vi "PlotDailies.vi"() -> ()   [LabVIEW 2019]
uses:
  <userlib>/LevyLab/XY Utilities/subVIs/Append (double array).vi
  <userlib>/LevyLab/XY Utilities/subVIs/Get X and Y (single).vi
  <userlib>/_OpenG.lib/array/array.llb/Sort 1D Array (DBL)__ogtk.vi
  <userlib>/_OpenG.lib/array/array.llb/Reorder 1D Array2 (Path)__ogtk.vi
  <userlib>/LevyLab/Graph Utilities/graph_utilities.lvclass
  <userlib>/LevyLab/XY Utilities/xy_utilities.lvlib
panel:
  in  "items":i32[](listbox)
  in  "files":i32[](listbox)
  out "XY Graph":cluster{dbl[], dbl[]}[](graph)
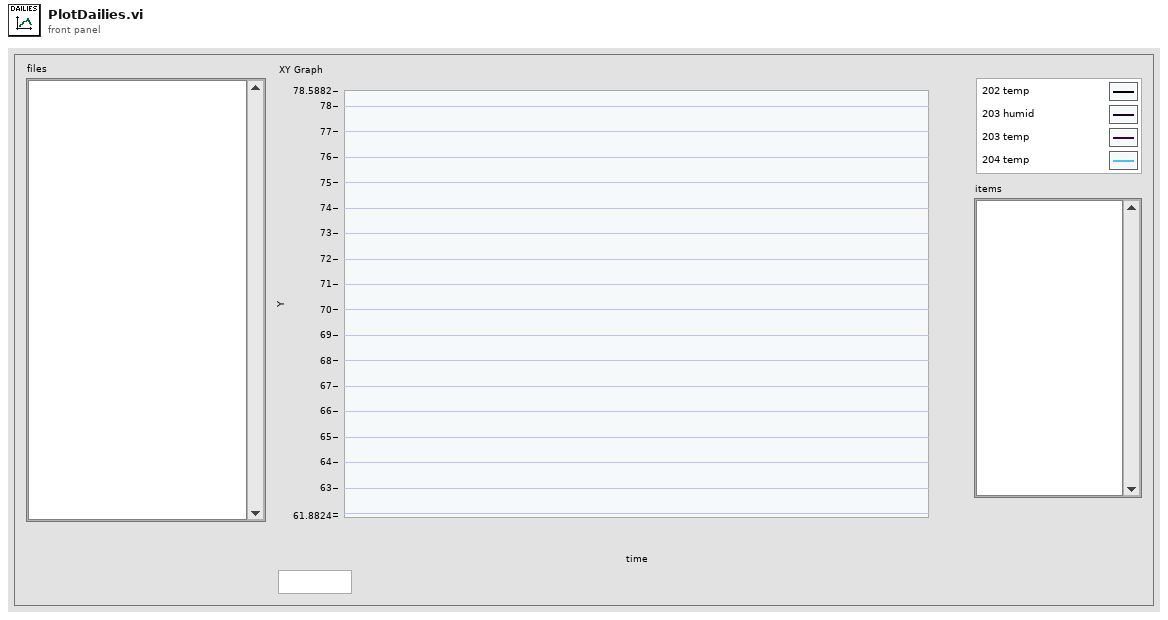
[diagram p1: front panel]
types:
  T1 = enum32{"Invalid", "Standard", "Closed", "Hidden", "Minimized", "Maximized"}
  T2 = enum32{"invalid app kind", "Development System", "Run Time System", "Student Edition", "Embedded LabVIEW", "Evaluation", "Custom"}
  T3 = enum16{"CET-C1", "CET-C1s", "CET-C2", "CET-C2s", "CET-C3", "CET-C3s", "CET-C4", "CET-C4s", "CET-C5", "CET-C5s", "CET-C6", "CET-C6s", "CET-C7", "CET-C7s", "CET-CBC1", "CET-CBC2", "CET-CBD1", "CET-CBL1", "CET-CBL2", "CET-D01", "CET-D01A", "CET-D02", "CET-D03", "CET-D04", "CET-D06", "CET-D07", "CET-D08", "CET-D09", "CET-D10", "CET-D11", "CET-D12", "CET-D13", "CET-I1", "CET-I2", "CET-I3", "CET-L01", "CET-L02", "CET-L03", "CET-L04", "CET-L05", "CET-L06", "CET-L07", "CET-L08", "CET-L09", "CET-L10", "CET-L11", "CET-L12", "CET-L13", "CET-L14", "CET-L15", "CET-L16", "CET-L17", "CET-L18", "CET-L19", "CET-L20", "CET-R1", "CET-R2", "CET-R3", "CET-R4"}
  T4 = enum16{"Inferno", "Kindlmann", "Plasma", "Viridis", "LevyLab2010", "ColorCET...", "Custom..."}
  T5 = cluster{"Core":cluster{"Current VI Reference":refnum<vi>, "Close Panel on Exit?":bool}, "dailies folder":path, "file paths":path[], "file path":path, "items":string[], "Map":map{string, dbl[]}, "XY-data":cluster{"X-array":dbl[], "Y-array":dbl[]}[]}
  T6 = cluster{"Current VI Reference":refnum<vi>, "Close Panel on Exit?":bool}
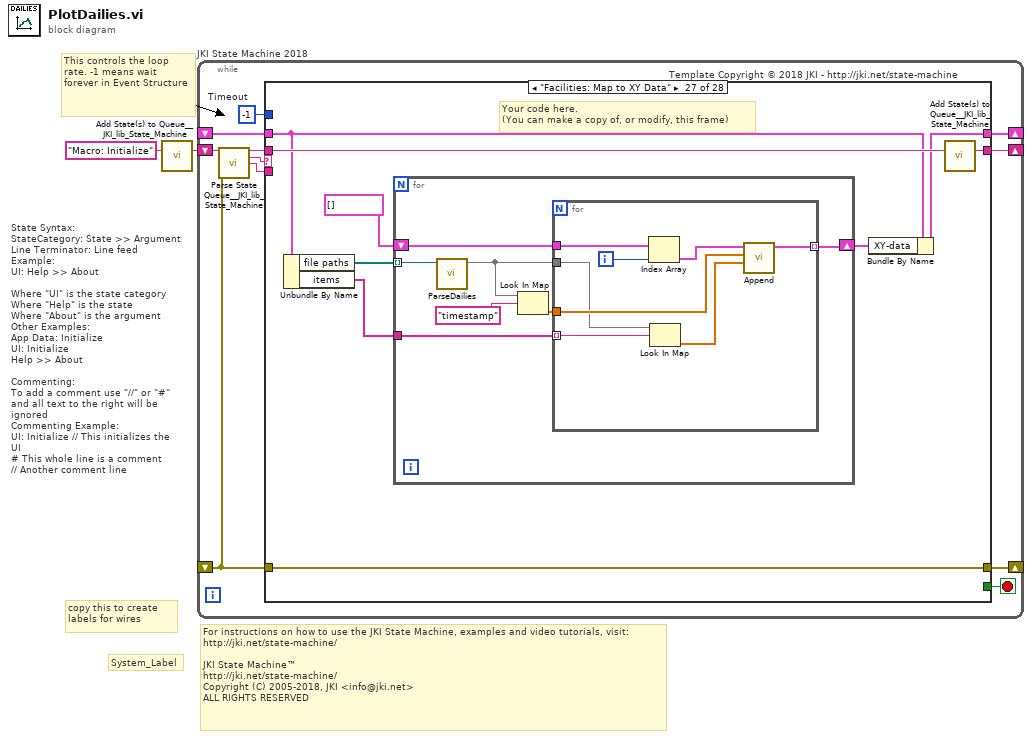
[diagram p0: block diagram]
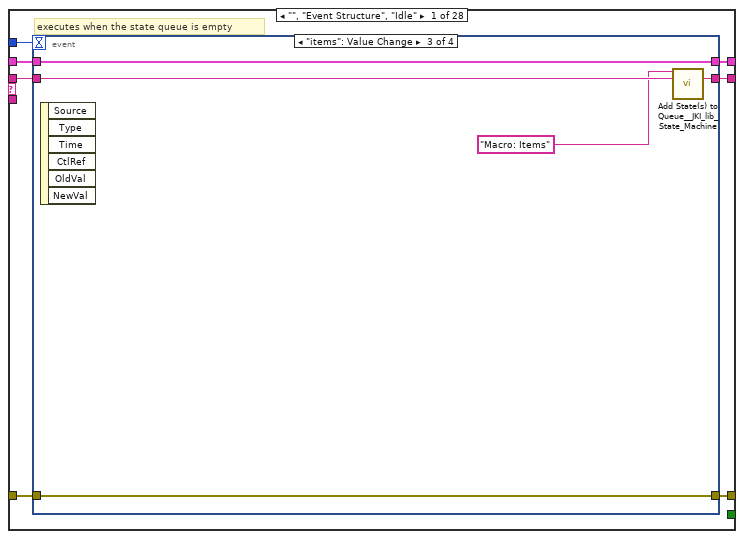
[diagram p2: hidden frame]
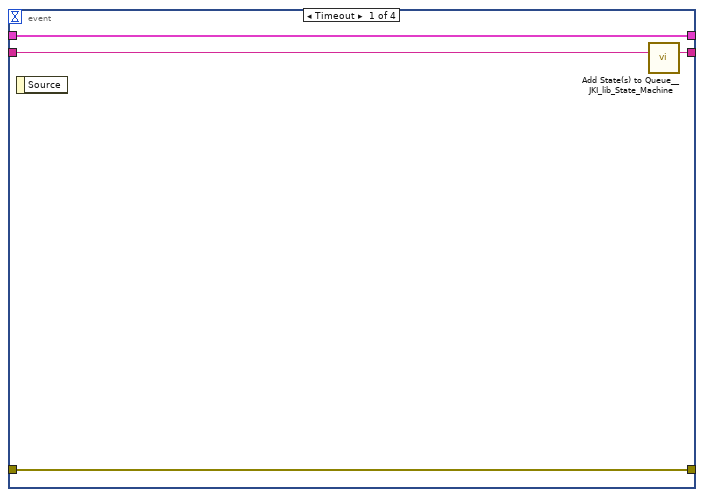
[diagram p3: hidden frame]
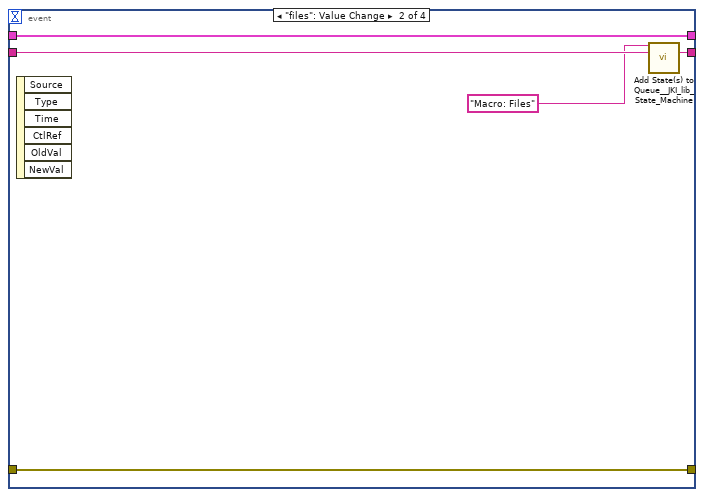
[diagram p4: hidden frame]
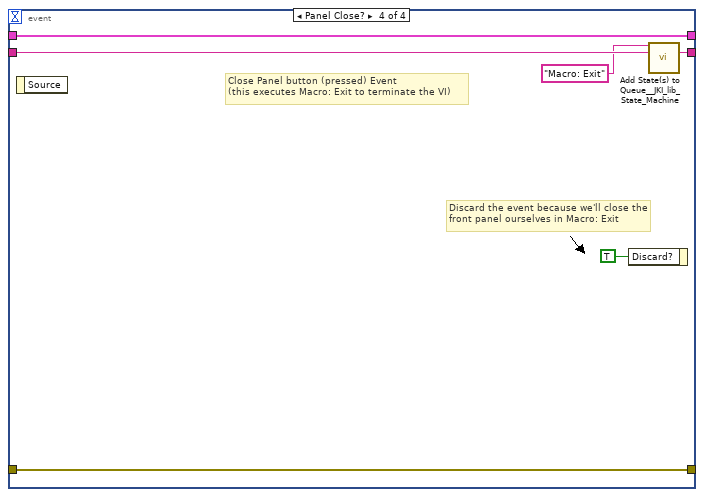
[diagram p5: hidden frame]
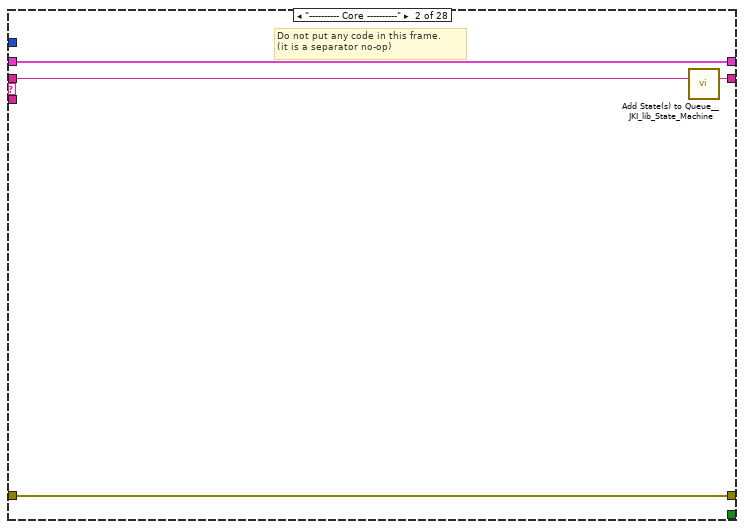
[diagram p6: hidden frame]
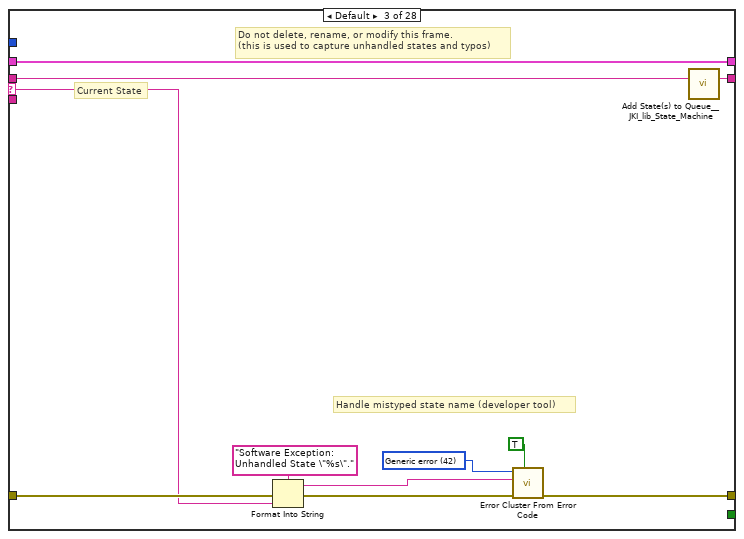
[diagram p7: hidden frame]
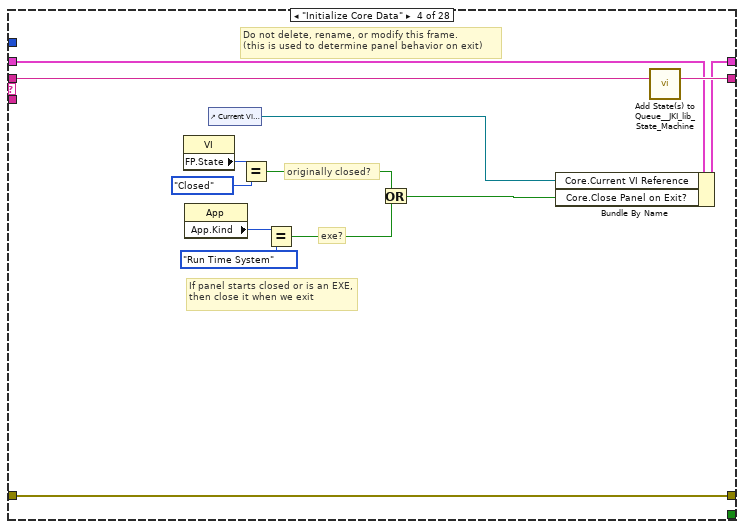
[diagram p8: hidden frame]
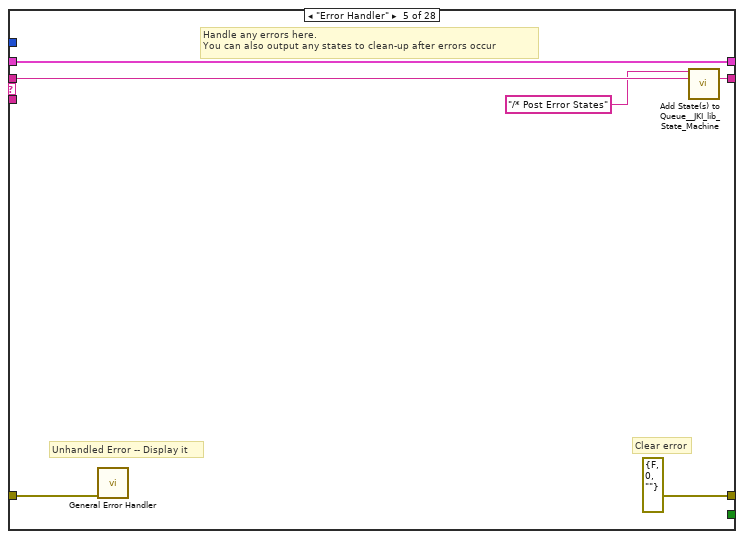
[diagram p9: hidden frame]
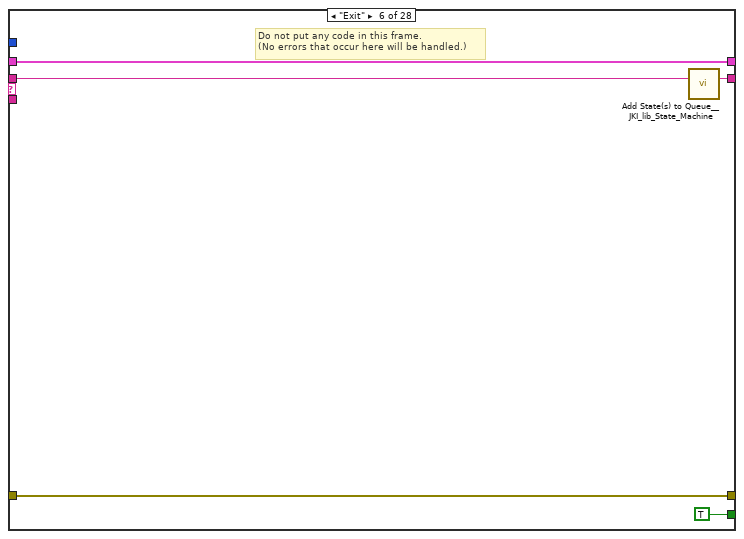
[diagram p10: hidden frame]
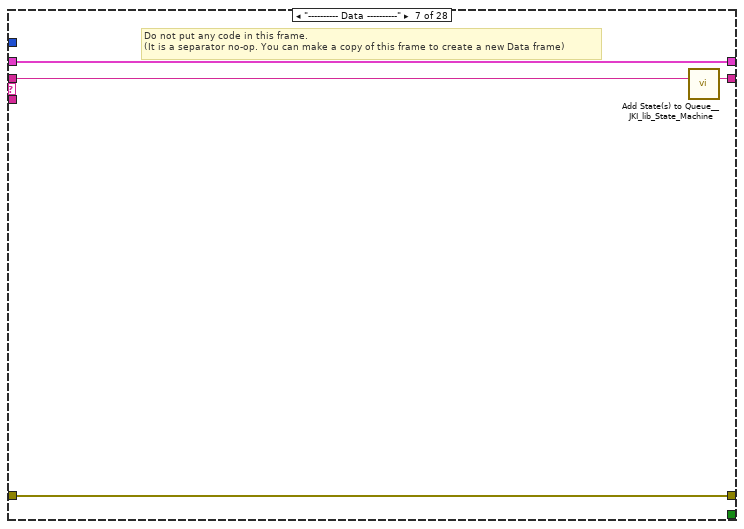
[diagram p11: hidden frame]
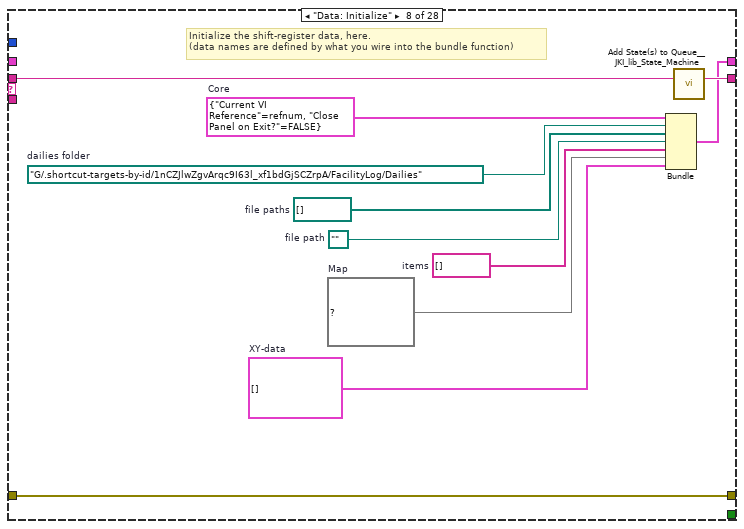
[diagram p12: hidden frame]
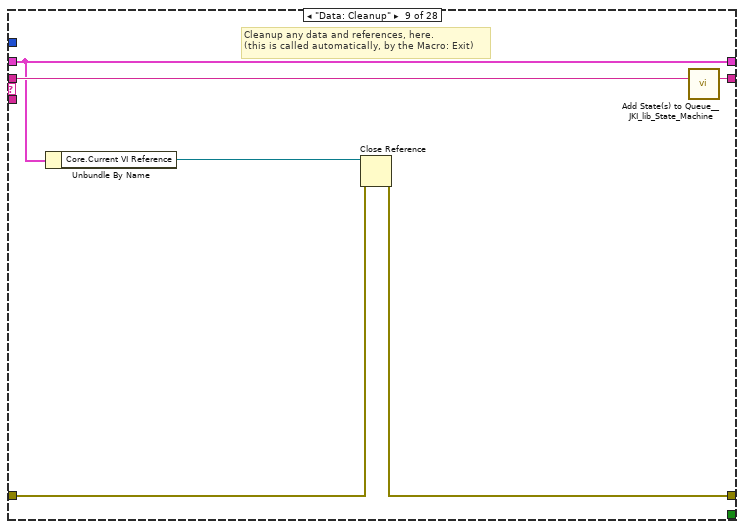
[diagram p13: hidden frame]
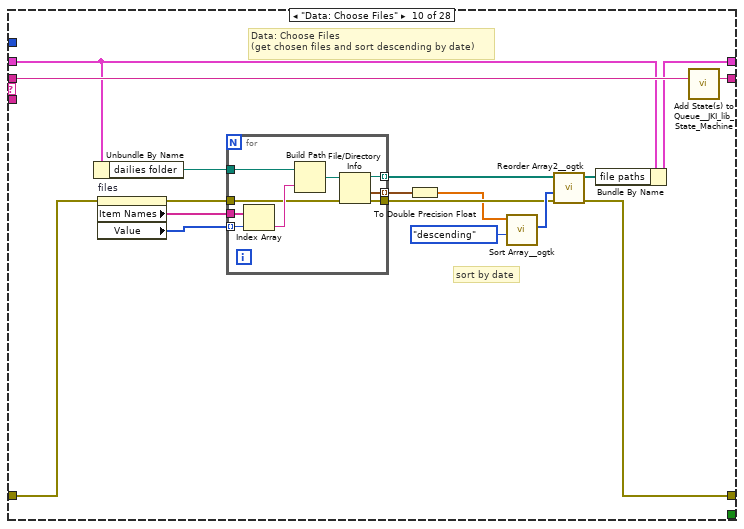
[diagram p14: hidden frame]
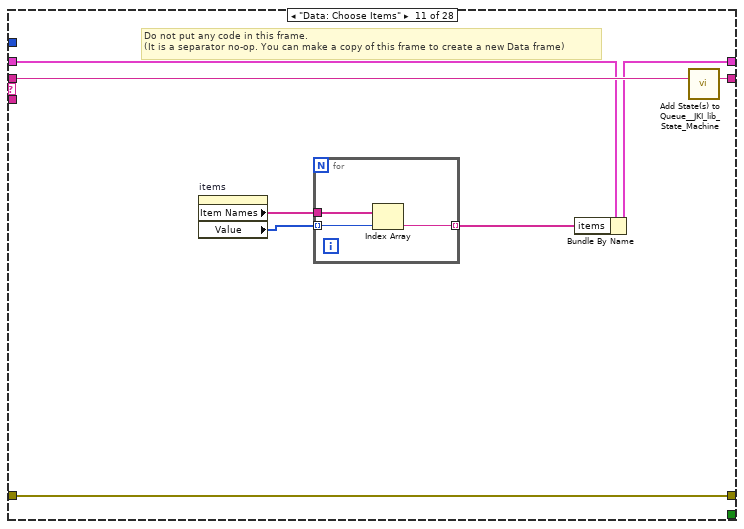
[diagram p15: hidden frame]
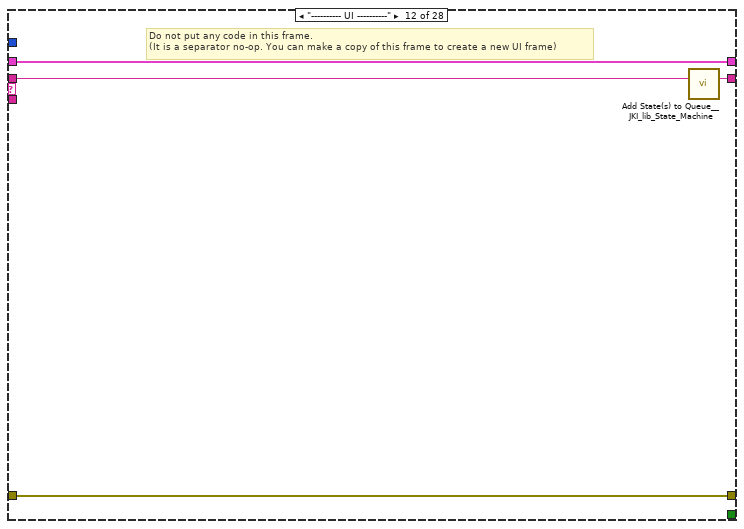
[diagram p16: hidden frame]
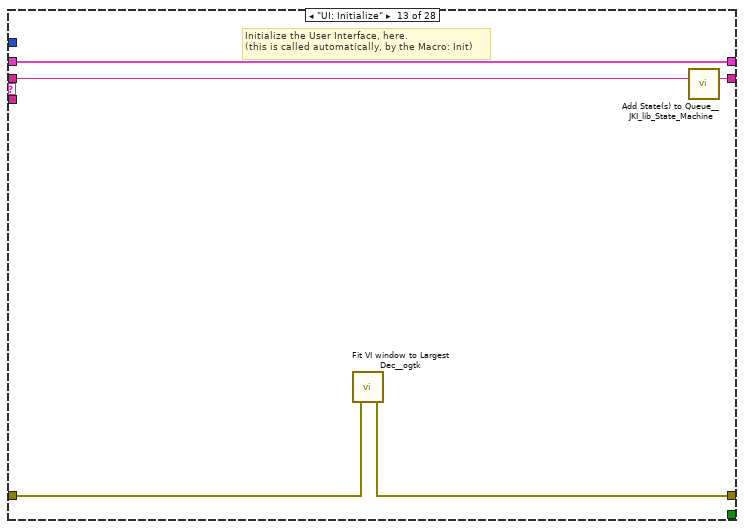
[diagram p17: hidden frame]
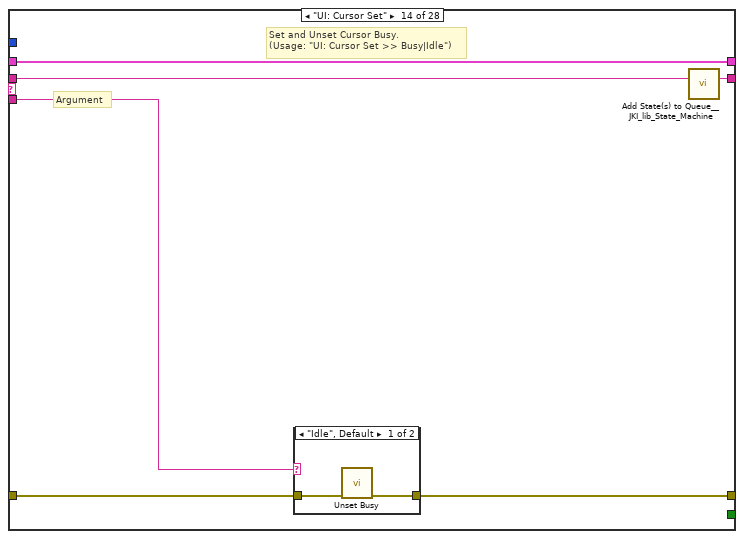
[diagram p18: hidden frame]
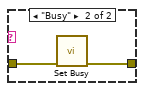
[diagram p19: hidden frame]
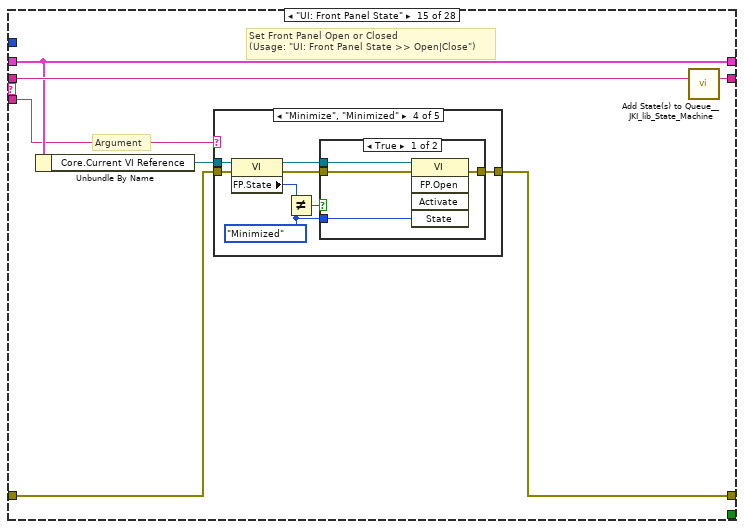
[diagram p20: hidden frame]
diagram:
  # "For instructions on how to use the JKI State Machine, examples and video tutorials, visit:\nhttp://jki.net/state-machine/\n\nJKI State Machine™\nhttp://jki.net/state-machine/\nCopyright (C) 2005-2018, JKI <info@jki.net>\nALL RIGHTS RESERVED"
  # "State Syntax:\nStateCategory: State >> Argument\nLine Terminator: Line feed\nExample:\nUI: Help >> About\n\nWhere \"UI\" is the state category\nWhere \"Help\" is the state\nWhere \"About\" is the argument\nOther Examples:\nApp Data: Initialize\nUI: Initialize\nHelp >> About\n\nCommenting:\nTo add a comment use \"//\" or \"#\" and all text to the right will be ignored\nCommenting Example:\nUI: Initialize // This initializes the UI\n# This whole line is a comment\n// Another comment line"
  # "copy this to create labels for wires"
  # "This controls the loop rate. -1 means wait forever in Event Structure"
  # "System_Label"
  n1 = call <vilib>:"Add State(s) to Queue__JKI_lib_State_Machine.vi"("State(s) in (\"\")"="Macro: Initialize") -> ("States Out"=w2:string)  [unwired: 14 in]
  n2 = while "JKI State Machine 2018" {
    shift-right: [w6] -> _
    shift-left: _ -> [w5]
    shift-right: [w9] -> _
    shift-left: _ -> [w3]
    shift-right: [w8] -> _
    shift-left: w2 -> [w10]
    stop <- w7 stop-if-true
    w4 = -1  # Timeout
    # "Template Copyright © 2018 JKI - http://jki.net/state-machine"
    n3 = call <vilib>:"Parse State Queue__JKI_lib_State_Machine.vi"("State Queue"=w10, "Error In (no error)"=w3) -> ("Remaining States"=w12:string, "Current State"=w13:string, "Arguments"=w11:string)  [unwired: 11 in]
    n4 = case shown="\"Facilities: Map to XY Data\"" w13 {
      selector: w13 -> [_ _ w45 _ _ _ _ _ _ _ _ _ _ _ _ _ _ _ _ _ _ _ _ _ _ _ _ _]
      tunnel: w12 -> [w20 w44 w49 w68 w74 w79 w83 w94 w100 w116 w133 w140 w145 w151 w162 w238 w244 w264 w278 w282 w288 w298 w309 w314 w318 w327 w336 w365]
      tunnel: w11 -> [_ _ _ _ _ _ _ _ _ _ _ _ _ w146 w156 _ _ _ _ _ _ _ _ _ _ _ _ _]
      tunnel: w5 -> [w18 w41 w47 w61 w71 w77 w80 _ w95 w101 w127 w137 w143 w149 w158 w232 w240 w261 w275 w279 w285 w295 w306 w311 w315 w325 w331 w355]
      tunnel: [w17 w42 w51 w65 errorcluster {"status"=FALSE, "code"=0, "source"=""} ("error out") w76 w81 w91 w96 w106 w131 w138 w142 w147 w159 w235 w242 w262 w276 w280 w286 w296 w307 w312 w316 w322 w334 w352] -> w9
      tunnel: w3 -> [w16 w42 w50 w65 w70 w76 w81 w91 w97 w105 w131 w138 w141 w148 w160 w234 w242 w262 w276 w280 w286 w296 w307 w312 w316 w321 w334 w353]
      tunnel: [w19 w43 w48 w67 w73 w78 w82 w93 w99 w115 w132 w139 w144 w150 w161 w237 w243 w263 w277 w281 w287 w297 w308 w313 w317 w326 w335 w364] -> w8
      tunnel: [_ _ _ _ _ TRUE _ _ _ _ _ _ _ _ _ _ _ _ _ _ _ _ _ _ _ _ _ _] -> w7
      tunnel: [w15 w41 w47 w66 w71 w77 w80 w92 w95 w102 w128 w137 w143 w149 w158 w232 w240 w261 w275 w279 w285 w295 w306 w311 w315 w323 w332 w356] -> w6
      tunnel: w4 -> [w14 _ _ _ _ _ _ _ _ _ _ _ _ _ _ _ _ _ _ _ _ _ _ _ _ _ _ _]
      frame "", "Event Structure", "Idle" {
        # "executes when the state queue is empty"
        n5 = event shown="[2] \"items\": Value Change" {
          selector: _ -> [_ _ _ _]
          dyn-events: _ -> [_ _ _ _]
          timeout: w14 -> [_ _ _ _]
          tunnel: w20 -> [w24 w29 w34 w40]
          tunnel: [w23 w28 w33 w39] -> w19
          tunnel: w18 -> [w21 w26 w31 w37]
          tunnel: [w22 w27 w32 w38] -> w17
          tunnel: w16 -> [w22 w27 w32 w38]
          tunnel: [w21 w26 w31 w37] -> w15
          event Timeout {
            n6 = event-data() -> ()  [unwired: 1 in, 1 out]
            n7 = call <vilib>:"Add State(s) to Queue__JKI_lib_State_Machine.vi"("State(s) in (\"\")"=w24) -> ("States Out"=w23:string)  [unwired: 14 in]
          }
          event "files": Value Change {
            n8 = event-data() -> ()  [unwired: 1 in, 6 out]
            n9 = call <vilib>:"Add State(s) to Queue__JKI_lib_State_Machine.vi"("State(s) in Front (\"\")"="Macro: Files" ("State(s) in Front (\"\")"), "State(s) in (\"\")"=w29) -> ("States Out"=w28:string)  [unwired: 13 in]
          }
          event "items": Value Change {
            n10 = event-data() -> ()  [unwired: 1 in, 6 out]
            n11 = call <vilib>:"Add State(s) to Queue__JKI_lib_State_Machine.vi"("State(s) in Front (\"\")"="Macro: Items" ("State(s) in Front (\"\")"), "State(s) in (\"\")"=w34) -> ("States Out"=w33:string)  [unwired: 13 in]
          }
          event Panel Close? {
            # "Discard the event because we'll close the front panel ourselves in Macro: Exit"
            # "Close Panel button (pressed) Event\n(this executes Macro: Exit to terminate the VI)"
            n12 = event-data() -> ()  [unwired: 1 in, 1 out]
            n13 = event-data("Discard?"=TRUE) -> ()  [unwired: 1 in, 1 out]
            n14 = call <vilib>:"Add State(s) to Queue__JKI_lib_State_Machine.vi"("State(s) in Front (\"\")"="Macro: Exit", "State(s) in (\"\")"=w40) -> ("States Out"=w39:string)  [unwired: 13 in]
          }
        }
      }
      frame "---------- Core ----------" {
        # "Do not put any code in this frame.\n(it is a separator no-op)"
        n15 = call <vilib>:"Add State(s) to Queue__JKI_lib_State_Machine.vi"("State(s) in (\"\")"=w44) -> ("States Out"=w43:string)  [unwired: 14 in]
      }
      frame Default {
        w54 = 42 items=["No error", "Argument error", "Memory is full", "Out of zone", "End of file", "File already open", "Generic file I/O error", "File not found", "File permission error", "Disk is full", "Duplicate path", "Too many files open", "System feature not enabled", "Resource file not found", "Cannot add resource", "Resource not found", "Image not found", "Image memory error", "Pen does not exist", "Config type invalid", "Config token not found", "Config parse error", "Config memory error", "Bad external code format", "Bad external code offset", "External code not present", "Null window", "Destroy window error", "Null menu", "Print aborted", "Bad print record", "Print driver error", "Windows error during printing", "Memory error during printing", "Print dialog error", "Generic print error", "Invalid device refnum", "Device not found", "Device parameter error", "Device unit error", "Cannot open device", "Device call aborted", "Generic error", "Cancelled by user", "Object ID too low", "Object ID too high", "Object not in heap", "Unknown heap", "Unknown object (invalid DefProc)", "Unknown object (DefProc not in table)", "Message out of range", "Invalid (null) method", "Unknown message", "Manager call not supported", "Bad address", "Network operation in progress", "Network operation timed out", "Connection is busy", "Network attribute not supported", "Network error", "Address in use", "System out of memory", "Connection aborted", "Connection refused", "Not connected", "Already connected", "Connection closed", "Initialization error (interapplication manager)", "Bad occurrence", "Wait on unbound occurrence handler", "Occurrence queue overflow", "Datalog type conflict", "Unused", "Unrecognized type (interapplication manager)", "Memory corrupt", "Failed to make temporary DLL", "Old CIN version", "Drag socket not found", "Failed to load drop-object", "Failed to register OLE object", "Failed to release OLE object", "Format specifier type mismatch", "Unknown format specifier", "Too few format specifiers", "Too many format specifiers", "Scan failed", "Newer CIN version", "Error converting to variant", "Runtime menu error", "Password tampered", "Variant attribute not found", "Incompatible variant data type", "Event data is not available", "Event Store is not present", "Occurrence is not found", "Event Queue is not created", "Event info is not available", "Refnum passed is NULL", "Error retrieving Class GUID", "Error retrieving CoClass GUID", "Error retrieving TypeLib GUID.", "Bad built application magic bytes.", "Specific driver is different from the specific driver associated with the Logical Name.", "There is no session opened to the class driver.", "Max Error", "MAX - Error with config objects", "MAX - Error loading configuration", "MAX - Group not supported"]
        # "Current State"
        # "Do not delete, rename, or modify this frame.\n(this is used to capture unhandled states and typos)"
        # "Handle mistyped state name (developer tool)"
        n16 = Format Into String(format string="Software Exception: Unhandled State \"%s\"." ("message"), error in=w50, w45) -> (resulting string=w53:string, error out=w52:errorcluster)  [unwired: 1 in]
        n17 = call <vilib>:"Error Cluster From Error Code.vi"("show call chain? (False)"=TRUE, "error in (no error)"=w52, "error message (\"\")"=w53, "error code (0)"=w54) -> ("error out"=w51:errorcluster)  [unwired: 5 in]
        n18 = call <vilib>:"Add State(s) to Queue__JKI_lib_State_Machine.vi"("State(s) in (\"\")"=w49) -> ("States Out"=w48:string)  [unwired: 14 in]
      }
      frame "Initialize Core Data" {
        # "Do not delete, rename, or modify this frame.\n(this is used to determine panel behavior on exit)"
        # "originally closed?"
        # "exe?"
        # "If panel starts closed or is an EXE, then close it when we exit"
        n19 = property class="VI"() -> ("FP.State"=w58:T1)  [unwired: 2 in, 2 out]
        n20 = property class="App"() -> ("App.Kind"=w64:T2)  [unwired: 2 in, 2 out]
        n21 = control-ref of="Current VI Reference"() -> (w59:refnum<vi>)
        n22 = Equal?(x=w58, y=T1."Closed" ("Front Panel Window:State")) -> (x = y?=w56:bool)
        n23 = Equal?(x=w64, y=T2."Run Time System" ("Application:Kind")) -> (x = y?=w62:bool)
        n24 = Or(x=w56, y=w62) -> (x .or. y?=w60:bool)
        n25 = Bundle By Name(cluster=w61, "Core.Current VI Reference"=w59, "Core.Close Panel on Exit?"=w60) -> (w66:T5)
        n26 = call <vilib>:"Add State(s) to Queue__JKI_lib_State_Machine.vi"("State(s) in (\"\")"=w68) -> ("States Out"=w67:string)  [unwired: 14 in]
      }
      frame "Error Handler" {
        # "Unhandled Error -- Display it"
        # "Handle any errors here.\nYou can also output any states to clean-up after errors occur"
        # "Clear error"
        n27 = call <vilib>:"General Error Handler.vi"("error in (no error)"=w70) -> ()  [unwired: 10 in, 5 out]
        n28 = call <vilib>:"Add State(s) to Queue__JKI_lib_State_Machine.vi"("State(s) in Front (\"\")"="/* Post Error States", "State(s) in (\"\")"=w74) -> ("States Out"=w73:string)  [unwired: 13 in]
      }
      frame "Exit" {
        # "Do not put any code in this frame.\n(No errors that occur here will be handled.)"
        n29 = call <vilib>:"Add State(s) to Queue__JKI_lib_State_Machine.vi"("State(s) in (\"\")"=w79) -> ("States Out"=w78:string)  [unwired: 14 in]
      }
      frame "---------- Data ----------" {
        # "Do not put any code in this frame.\n(It is a separator no-op. You can make a copy of this frame to create a new Data frame)"
        n30 = call <vilib>:"Add State(s) to Queue__JKI_lib_State_Machine.vi"("State(s) in (\"\")"=w83) -> ("States Out"=w82:string)  [unwired: 14 in]
      }
      frame "Data: Initialize" {
        w84 = string[] []  # items
        w85 = cluster{"X-array":dbl[], "Y-array":dbl[]}[] []  # XY-data
        w86 = path[] []  # file paths
        w87 = path "G:/.shortcut-targets-by-id/1nCZJlwZgvArqc9I63l_xf1bdGjSCZrpA/FacilityLog/Dailies"  # dailies folder
        w88 = map{string, dbl[]} {}  # Map
        w89 = path ""  # file path
        w90 = T6 {"Current VI Reference"=refnum, "Close Panel on Exit?"=FALSE}  # Core
        # "Initialize the shift-register data, here.\n(data names are defined by what you wire into the bundle function)"
        n31 = Bundle("Core"=w90, "dailies folder"=w87, "file paths"=w86, "file path"=w89, "items"=w84, "Map"=w88, "XY-data"=w85) -> (w92:T5)  [unwired: 1 in]
        n32 = call <vilib>:"Add State(s) to Queue__JKI_lib_State_Machine.vi"("State(s) in (\"\")"=w94) -> ("States Out"=w93:string)  [unwired: 14 in]
      }
      frame "Data: Cleanup" {
        # "Cleanup any data and references, here.\n(this is called automatically, by the Macro: Exit)"
        n33 = Unbundle By Name(w95) -> ("Core.Current VI Reference"=w98:refnum<vi>)
        n34 = Close Reference(reference=w98, error in (no error)=w97) -> (error out=w96:errorcluster)
        n35 = call <vilib>:"Add State(s) to Queue__JKI_lib_State_Machine.vi"("State(s) in (\"\")"=w100) -> ("States Out"=w99:string)  [unwired: 14 in]
      }
      frame "Data: Choose Files" {
        # "sort by date"
        # "Data: Choose Files\n(get chosen files and sort descending by date)"
        n36 = Unbundle By Name(w101) -> ("dailies folder"=w112:path)
        n37 = property on="files" class="LstBox (strict)"(error in=w105) -> (error out=w107:errorcluster, "Item Names"=w114:string[], "Value"=w113:i32[])  [unwired: 1 in, 1 out]
        n38 = for {
          tunnel: w112 -> [w120]
          tunnel: [w125] -> w108 mode=indexing
          tunnel: [w124] -> w109 mode=indexing
          tunnel: w113 -> [w123] mode=indexing
          tunnel: w114 -> [w122]
          tunnel: [w118] -> w106
          tunnel: w107 -> [w117]
          n39 = Index Array(array=w122, index=w123) -> (element=w121:string)
          n40 = Build Path(base path=w120, name or relative path=w121) -> (appended path=w119:path)
          n41 = File/Directory Info(path=w119, error in=w117) -> (path out=w124:path, last mod=w125:timestamp, error out=w118:errorcluster)  [unwired: 4 out]
        }
        n42 = To Double Precision Float(number=w108) -> (double precision float=w104:dbl[])
        n43 = call-poly <userlib>:"Sort Array__ogtk.vi"("Order"=enum16{"ascending", "descending"}."descending", "Array in"=w104) -> ("Sorted Pointers"=w110:i32[])  [unwired: 8 in, 1 out]
        n44 = call-poly <userlib>:"Reorder Array2__ogtk.vi"("indices"=w110, "array"=w109) -> ("reordered array"=w103:path[])  [unwired: 9 in]
        n45 = Bundle By Name(cluster=w101, "file paths"=w103) -> (w102:T5)
        n46 = call <vilib>:"Add State(s) to Queue__JKI_lib_State_Machine.vi"("State(s) in (\"\")"=w116) -> ("States Out"=w115:string)  [unwired: 14 in]
      }
      frame "Data: Choose Items" {
        # "Do not put any code in this frame.\n(It is a separator no-op. You can make a copy of this frame to create a new Data frame)"
        n47 = property on="items" class="LstBox (strict)"() -> ("Item Names"=w130:string[], "Value"=w129:i32[])  [unwired: 2 in, 2 out]
        n48 = for {
          tunnel: w130 -> [w136]
          tunnel: w129 -> [w135] mode=indexing
          tunnel: [w134] -> w126 mode=indexing
          n49 = Index Array(array=w136, index=w135) -> (element=w134:string)
        }
        n50 = Bundle By Name(cluster=w127, "items"=w126) -> (w128:T5)
        n51 = call <vilib>:"Add State(s) to Queue__JKI_lib_State_Machine.vi"("State(s) in (\"\")"=w133) -> ("States Out"=w132:string)  [unwired: 14 in]
      }
      frame "---------- UI ----------" {
        # "Do not put any code in this frame.\n(It is a separator no-op. You can make a copy of this frame to create a new UI frame)"
        n52 = call <vilib>:"Add State(s) to Queue__JKI_lib_State_Machine.vi"("State(s) in (\"\")"=w140) -> ("States Out"=w139:string)  [unwired: 14 in]
      }
      frame "UI: Initialize" {
        # "Initialize the User Interface, here.\n(this is called automatically, by the Macro: Init)"
        n53 = call <userlib>:"Fit VI window to Largest Dec__ogtk.vi"("error in (no error)"=w141) -> ("error out"=w142:errorcluster)  [unwired: 5 in, 1 out]
        n54 = call <vilib>:"Add State(s) to Queue__JKI_lib_State_Machine.vi"("State(s) in (\"\")"=w145) -> ("States Out"=w144:string)  [unwired: 14 in]
      }
      frame "UI: Cursor Set" {
        # "Argument"
        # "Set and Unset Cursor Busy.\n(Usage: \"UI: Cursor Set >> Busy|Idle\")"
        n55 = case shown="\"Idle\", Default" w146 {
          tunnel: w148 -> [w153 w155]
          tunnel: [w152 w154] -> w147
          frame "Idle", Default {
            n56 = call <vilib>:"Unset Busy.vi"("error in (no error)"=w153) -> ("error out"=w152:errorcluster)  [unwired: 10 in]
          }
          frame "Busy" {
            n57 = call <vilib>:"Set Busy.vi"("error in (no error)"=w155) -> ("error out"=w154:errorcluster)  [unwired: 9 in, 1 out]
          }
        }
        n58 = call <vilib>:"Add State(s) to Queue__JKI_lib_State_Machine.vi"("State(s) in (\"\")"=w151) -> ("States Out"=w150:string)  [unwired: 14 in]
      }
      frame "UI: Front Panel State" {
        # "Argument"
        # "Set Front Panel Open or Closed\n(Usage: \"UI: Front Panel State >> Open|Close\")"
        n59 = Unbundle By Name(w158) -> ("Core.Current VI Reference"=w157:refnum<vi>)
        n60 = case shown="\"Minimize\", \"Minimized\"" w156 {
          tunnel: w160 -> [w168 w183 w194 w207 w220]
          tunnel: [w170 w184 w196 w209 w222] -> w159
          tunnel: w157 -> [w169 w181 w195 w208 w221]
          frame "Open", "Standard", Default {
            w163 = T1."Standard" ("State")
            n61 = property class="VI"(reference=w169, error in=w168) -> (reference out=w166:refnum<vi>, error out=w167:errorcluster, "FP.State"=w165:T1)
            n62 = Not Equal?(x=w165, y=w163) -> (x != y?=w164:bool)
            n63 = case shown="True" w164 {
              tunnel: [w174 w176] -> w170
              tunnel: w167 -> [w173 w176]
              tunnel: w166 -> [w172 _]
              tunnel: w163 -> [w171 _]
              frame True {
                n64 = invoke class="VI" method="FP.Open"(reference=w172, error in=w173, "Activate"=TRUE, "State"=w171) -> (error out=w174:errorcluster)  [unwired: 1 in, 4 out]
              }
              frame False {
              }
            }
          }
          frame "Close", "Closed" {
            n65 = property class="VI"(reference=w181, error in=w183) -> (reference out=w180:refnum<vi>, error out=w182:errorcluster, "FP.State"=w178:T1)
            n66 = Not Equal?(x=w178, y=T1."Closed" ("Front Panel Window:State")) -> (x != y?=w177:bool)
            n67 = case shown="True" w177 {
              tunnel: [w185 w188] -> w184
              tunnel: w182 -> [w185 w187]
              tunnel: w180 -> [_ w186]
              frame False {
              }
              frame True {
                n68 = invoke class="VI" method="FP.Close"(reference=w186, error in=w187) -> (error out=w188:errorcluster)  [unwired: 1 in, 2 out]
              }
            }
          }
          frame "Hidden", "Hide" {
            w189 = T1."Hidden" ("State")
            n69 = property class="VI"(reference=w195, error in=w194) -> (reference out=w192:refnum<vi>, error out=w193:errorcluster, "FP.State"=w191:T1)
            n70 = Not Equal?(x=w191, y=w189) -> (x != y?=w190:bool)
            n71 = case shown="True" w190 {
              tunnel: [w200 w201] -> w196
              tunnel: w193 -> [w199 w201]
              tunnel: w192 -> [w198 _]
              tunnel: w189 -> [w197 _]
              frame True {
                n72 = invoke class="VI" method="FP.Open"(reference=w198, error in=w199, "State"=w197) -> (error out=w200:errorcluster)  [unwired: 2 in, 4 out]
              }
              frame False {
              }
            }
          }
          frame "Minimize", "Minimized" {
            w202 = T1."Minimized" ("State")
            n73 = property class="VI"(reference=w208, error in=w207) -> (reference out=w205:refnum<vi>, error out=w206:errorcluster, "FP.State"=w204:T1)
            n74 = Not Equal?(x=w204, y=w202) -> (x != y?=w203:bool)
            n75 = case shown="True" w203 {
              tunnel: [w213 w214] -> w209
              tunnel: w206 -> [w212 w214]
              tunnel: w205 -> [w211 _]
              tunnel: w202 -> [w210 _]
              frame True {
                n76 = invoke class="VI" method="FP.Open"(reference=w211, error in=w212, "State"=w210) -> (error out=w213:errorcluster)  [unwired: 2 in, 4 out]
              }
              frame False {
              }
            }
          }
          frame "Maximize", "Maximized" {
            w215 = T1."Maximized" ("State")
            n77 = property class="VI"(reference=w221, error in=w220) -> (reference out=w218:refnum<vi>, error out=w219:errorcluster, "FP.State"=w217:T1)
            n78 = Not Equal?(x=w217, y=w215) -> (x != y?=w216:bool)
            n79 = case shown="True" w216 {
              tunnel: [w226 w227] -> w222
              tunnel: w219 -> [w225 w227]
              tunnel: w218 -> [w224 _]
              tunnel: w215 -> [w223 _]
              frame True {
                n80 = invoke class="VI" method="FP.Open"(reference=w224, error in=w225, "State"=w223) -> (error out=w226:errorcluster)  [unwired: 2 in, 4 out]
              }
              frame False {
              }
            }
          }
        }
        n81 = call <vilib>:"Add State(s) to Queue__JKI_lib_State_Machine.vi"("State(s) in (\"\")"=w162) -> ("States Out"=w161:string)  [unwired: 14 in]
      }
      frame "UI: Update File List" {
        # "put items into listbox"
        # "list *.csv files"
        # "UI: Update File List\n(list csv files and populate listbox)"
        n82 = Unbundle By Name(w232) -> ("dailies folder"=w231:path)
        n83 = List Folder(path=w231, pattern="*.csv", error in=w234) -> (filenames=w230:string[], error out=w236:errorcluster)  [unwired: 1 in, 2 out]
        n84 = Sort 1D Array(array=w230) -> (sorted array=w229:string[])
        n85 = Reverse 1D Array(array=w229) -> (reversed array=w228:string[])
        n86 = property on="files" class="LstBox (strict)"(error in=w236, "Item Names"=w228) -> (error out=w235:errorcluster)  [unwired: 1 in, 1 out]
        n87 = call <vilib>:"Add State(s) to Queue__JKI_lib_State_Machine.vi"("State(s) in (\"\")"=w238) -> ("States Out"=w237:string)  [unwired: 14 in]
      }
      frame "UI: Update Items" {
        # "Do not put any code in this frame.\n(It is a separator no-op. You can make a copy of this frame to create a new UI frame)"
        n88 = Unbundle By Name(w240) -> ("Map"=w239:map{string, dbl[]})
        n89 = for {
          tunnel: w239 -> [w246] mode=indexing
          tunnel: [w245] -> w241 mode=indexing
          n90 = Unbundle(w246) -> (w245:string)  [unwired: 1 out]
        }
        n91 = property on="items" class="LstBox (strict)"("Item Names"=w241) -> ()  [unwired: 2 in, 2 out]
        n92 = call <vilib>:"Add State(s) to Queue__JKI_lib_State_Machine.vi"("State(s) in (\"\")"=w244) -> ("States Out"=w243:string)  [unwired: 14 in]
      }
      frame "UI: Update Graph Legend" {
        w247 = u8 0 ("Plot.Point Style")
        # "Do not put any code in this frame.\n(It is a separator no-op. You can make a copy of this frame to create a new UI frame)"
        n93 = property on="items" class="LstBox (strict)" props=["Value", "Item Names", "Value"]() -> ("Item Names"=w258:string[], "Value"=w256:i32[])  [unwired: 2 in, 3 out]
        n94 = Array Size(array=w256) -> (size(s)=w259:i32)
        n95 = call <userlib>:"Choose Color Table.vi"("Size (256)"=w259, "ColorCET"=T3."CET-I3", "Color Map"=T4."ColorCET...") -> ("Color Table"=w257:u32[])  [unwired: 5 in, 3 out]
        n96 = for {
          tunnel: w258 -> [w273]
          tunnel: w256 -> [w272] mode=indexing
          tunnel: w257 -> [w266] mode=indexing
          tunnel: [w265] -> w250
          i -> [w265]
          n97 = Index Array(array=w273, index=w272) -> (element=w268:string)
          n98 = property on="XY Graph" class="XYGraph (strict)"("Active Plot"=w265, "Plot.Plot Name"=w268, "Plot.Bar Plot Style"=u8 0, "Plot.Line Style"=u8 0, "Plot.Point Style"=u8 5, "Plot.Fill/Pt. Color"=w266, "Plot.Line Width"=u8 0) -> ()  [unwired: 2 in, 2 out]
        }
        n99 = Increment(x=w250) -> (x+1=w248:i32)
        n100 = property on="XY Graph" class="XYGraph (strict)"("Active Plot"=w248, "Plot.Plot Name"="weekend", "Plot.Bar Plot Style"=u8 2, "Plot.Fill To"=i16 -2, "Plot.Point Style"=u8 0, "Plot.Fill/Pt. Color"=u32 16771047, "Plot.Line Style"=w247, "Plot.Line Width"=w247) -> ()  [unwired: 2 in, 2 out]
        n101 = call <vilib>:"Add State(s) to Queue__JKI_lib_State_Machine.vi"("State(s) in (\"\")"=w264) -> ("States Out"=w263:string)  [unwired: 14 in]
      }
      frame "UI: Update Graph" {
        # "Do not put any code in this frame.\n(It is a separator no-op. You can make a copy of this frame to create a new UI frame)"
        n102 = Unbundle By Name(w275) -> ("XY-data"=→"XY Graph":cluster{"X-array":dbl[], "Y-array":dbl[]}[])
        n103 = call <vilib>:"Add State(s) to Queue__JKI_lib_State_Machine.vi"("State(s) in (\"\")"=w278) -> ("States Out"=w277:string)  [unwired: 14 in]
      }
      frame "---------- Macro ----------" {
        # "Do not put any code in this frame.\n(It is a separator no-op. You can make a copy of this frame to create a new Macro frame)"
        n104 = call <vilib>:"Add State(s) to Queue__JKI_lib_State_Machine.vi"("State(s) in (\"\")"=w282) -> ("States Out"=w281:string)  [unwired: 14 in]
      }
      frame "Macro: Initialize" {
        w284 = "Data: Initialize\nInitialize Core Data\nUI: Initialize\nUI: Front Panel State >> Open"  # Data: Initialize Initialize Core Data UI: Initialize UI: Front Panel State >> Open
        # "Initialization Macro\n(This is called once, when the VI starts)"
        n105 = call <vilib>:"Add State(s) to Queue__JKI_lib_State_Machine.vi"("State(s) in Front (\"\")"=w284, "State(s) in (\"\")"=w288, "State(s) at Back (\"\")"="UI: Update File List") -> ("States Out"=w287:string)  [unwired: 12 in]
      }
      frame "Macro: Exit" {
        # "Exit Macro\n(This is called once, when the VI exits)"
        n106 = Unbundle By Name(w295) -> ("Core.Close Panel on Exit?"=w294:bool)
        n107 = Select(t="UI: Front Panel State >> Close", s=w294, f="") -> (s? t:f=w291:string)
        n108 = call <vilib>:"Add State(s) to Queue__JKI_lib_State_Machine.vi"("State(s) in (\"\")"=w291, "State(s) at Back (\"\")"="Data: Cleanup\nExit") -> ("States Out"=w289:string)  [unwired: 13 in]
        n109 = call <vilib>:"Add State(s) to Queue__JKI_lib_State_Machine.vi"("State(s) in Front (\"\")"=w289, "State(s) in (\"\")"=w298) -> ("States Out"=w297:string)  [unwired: 13 in]
      }
      frame "Macro: Files" {
        # "Do not put any code in this frame.\n(It is a separator no-op. You can make a copy of this frame to create a new Macro frame)"
        n110 = Unbundle By Name(w306) -> ("items"=w305:string[])
        n111 = Empty Array?(array=w305) -> (empty?=w304:bool)
        n112 = Select(t="" ("State(s) in Front (\"\")"), s=w304, f="Macro: Items" ("State(s) in Front (\"\")")) -> (s? t:f=w301:string)
        n113 = call <vilib>:"Add State(s) to Queue__JKI_lib_State_Machine.vi"("State(s) in Front (\"\")"="Data: Choose Files\nFacilities: Read CSV\nUI: Update Items" ("State(s) in Front (\"\")"), "State(s) at Back (\"\")"=w301) -> ("States Out"=w299:string)  [unwired: 13 in]
        n114 = call <vilib>:"Add State(s) to Queue__JKI_lib_State_Machine.vi"("State(s) in Front (\"\")"=w299, "State(s) in (\"\")"=w309) -> ("States Out"=w308:string)  [unwired: 13 in]
      }
      frame "Macro: Items" {
        # "Do not put any code in this frame.\n(It is a separator no-op. You can make a copy of this frame to create a new Macro frame)"
        n115 = call <vilib>:"Add State(s) to Queue__JKI_lib_State_Machine.vi"("State(s) in Front (\"\")"="Data: Choose Items\nUI: Update Graph Legend\nFacilities: Map to XY Data\nFacilities: Create Weekend Trace\nUI: Update Graph" ("State(s) in Front (\"\")"), "State(s) in (\"\")"=w314) -> ("States Out"=w313:string)  [unwired: 13 in]
      }
      frame "---------- Facilities ----------" {
        # "Template Separator\n(You can make a copy of, or modify, this frame)"
        n116 = call <vilib>:"Add State(s) to Queue__JKI_lib_State_Machine.vi"("State(s) in (\"\")"=w318) -> ("States Out"=w317:string)  [unwired: 14 in]
      }
      frame "Facilities: Read CSV" {
        # "Your code here.\n(You can make a copy of, or modify, this frame)"
        n117 = Unbundle By Name(w325) -> ("file paths"=w320:path[])
        n118 = Index Array(array=w320) -> (element=w319:path)  [unwired: 1 in]
        n119 = call "ParseDailies.vi"("error in (no error)"=w321, "file path in"=w319) -> ("error out"=w322:errorcluster, "Map"=w324:map{string, dbl[]})  [unwired: 8 in]
        n120 = Bundle By Name(cluster=w325, "Map"=w324) -> (w323:T5)
        n121 = call <vilib>:"Add State(s) to Queue__JKI_lib_State_Machine.vi"("State(s) in (\"\")"=w327) -> ("States Out"=w326:string)  [unwired: 14 in]
      }
      frame "Facilities: Map to XY Data" {
        # "Your code here.\n(You can make a copy of, or modify, this frame)"
        n122 = Unbundle By Name(w331) -> ("file paths"=w329:path[], "items"=w330:string[])
        n123 = for {
          tunnel: w330 -> [w338]
          tunnel: w329 -> [w337] mode=indexing
          shift-right: [w340] -> w333
          shift-left: cluster{"X-array":dbl[], "Y-array":dbl[]}[] [] -> [w342]
          n124 = call "ParseDailies.vi"("file path in"=w337) -> ("Map"=w339:map{string, dbl[]})  [unwired: 9 in, 1 out]
          n125 = Look In Map(map=w339, key="timestamp") -> (value=w341:dbl[])  [unwired: 1 in, 1 out]
          n126 = for {
            tunnel: w342 -> [w351]
            tunnel: w339 -> [w344]
            tunnel: w341 -> [w346]
            tunnel: [w348] -> w340 mode=indexing
            tunnel: w338 -> [w345] mode=indexing
            i -> [w350]
            n127 = Index Array(array=w351, index=w350) -> (element=w349:cluster{"X-array":dbl[], "Y-array":dbl[]})
            n128 = Look In Map(map=w344, key=w345) -> (value=w347:dbl[])  [unwired: 1 in, 1 out]
            n129 = call-poly <userlib>:"Append.vi"("Y-array"=w347, "X-array"=w346, "XY-data (A)"=w349) -> ("XY-data out"=w348:cluster{"X-array":dbl[], "Y-array":dbl[]})  [unwired: 7 in, 1 out]
          }
        }
        n130 = Bundle By Name(cluster=w331, "XY-data"=w333) -> (w332:T5)
        n131 = call <vilib>:"Add State(s) to Queue__JKI_lib_State_Machine.vi"("State(s) in (\"\")"=w336) -> ("States Out"=w335:string)  [unwired: 14 in]
      }
      frame "Facilities: Create Weekend Trace" {
        # "Template Separator\n(You can make a copy of, or modify, this frame)"
        n132 = Unbundle By Name(w355) -> ("XY-data"=w362:cluster{"X-array":dbl[], "Y-array":dbl[]}[])
        n133 = Index Array(array=w362) -> (element=w360:cluster{"X-array":dbl[], "Y-array":dbl[]})  [unwired: 1 in]
        n134 = call-poly <userlib>:"Get X and Y.vi"("error in (no error)"=w353, "XY-data"=w360) -> ("error out"=w354:errorcluster, "X-array"=w357:dbl[])  [unwired: 6 in, 2 out]
        n135 = To Time Stamp(1:w357) -> (0:w363:timestamp[])
        n136 = for {
          tunnel: w363 -> [w373] mode=indexing
          tunnel: [w366] -> w359 mode=indexing
          n137 = Format Into String(format string="%<%A>T", w373) -> (resulting string=w370:string)  [unwired: 2 in, 1 out]
          n138 = call <userlib>:"MGI String Pattern Match Exists.vi"("Patterns to Try"=string[] ["Saturday", "Sunday"], "String"=w370) -> ("Match Found"=w369:bool)  [unwired: 1 out]
          n139 = Select(t=100.0, s=w369, f=0.0) -> (s? t:f=w366:dbl)
        }
        n140 = call <userlib>:"Initialize.vi"("error in (no error)"=w354, "Y-array"=w359, "X-array"=w357) -> ("error out"=w352:errorcluster, "XY-data out"=w358:cluster{"X-array":dbl[], "Y-array":dbl[]})  [unwired: 7 in]
        n141 = Build Array (concatenate)(w362, w358) -> (w361:cluster{"X-array":dbl[], "Y-array":dbl[]}[])
        n142 = Bundle By Name(cluster=w355, "XY-data"=w361) -> (w356:T5)
        n143 = call <vilib>:"Add State(s) to Queue__JKI_lib_State_Machine.vi"("State(s) in (\"\")"=w365) -> ("States Out"=w364:string)  [unwired: 14 in]
      }
    }
  }
